vi "Quick Scale.vi"   [LabVIEW 2024, in "NI_AALBase.lvlib"]
doc: "<p>Determines the maximum absolute value of the input <strong>X</strong> and then scales <strong>X</strong> using this value.</p>"
uses:
  NI_AALBase.lvlib
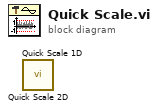
[diagram p0: block diagram]
diagram:
  n1 = call "Quick Scale 2D.vi"() -> ()  [unwired: 1 in, 3 out]
  n2 = call "Quick Scale 1D.vi"() -> ()  [unwired: 1 in, 3 out]
